vi "Read current data.vi"(8 "error in":errorcluster) -> (0 "error out":errorcluster, 1 "timestamp":timestamp, 2 "Data Array":T1[](array[typedef]), 3 "Variable Descriptions":T2[](array[typedef]))   [LabVIEW 2017, in "DTACQ - Network Enabled Device Driver.lvlib"]
uses:
  DTACQ - Network Enabled Device Driver.lvlib
  Network Shared Variables/Typedefs/Shared Variable Properties--Cluster.ctl
  Network Shared Variables/Typedefs/X and Y Variant Arrays--Cluster.ctl
  Network Shared Variables/Shared Variables Library.lvlib
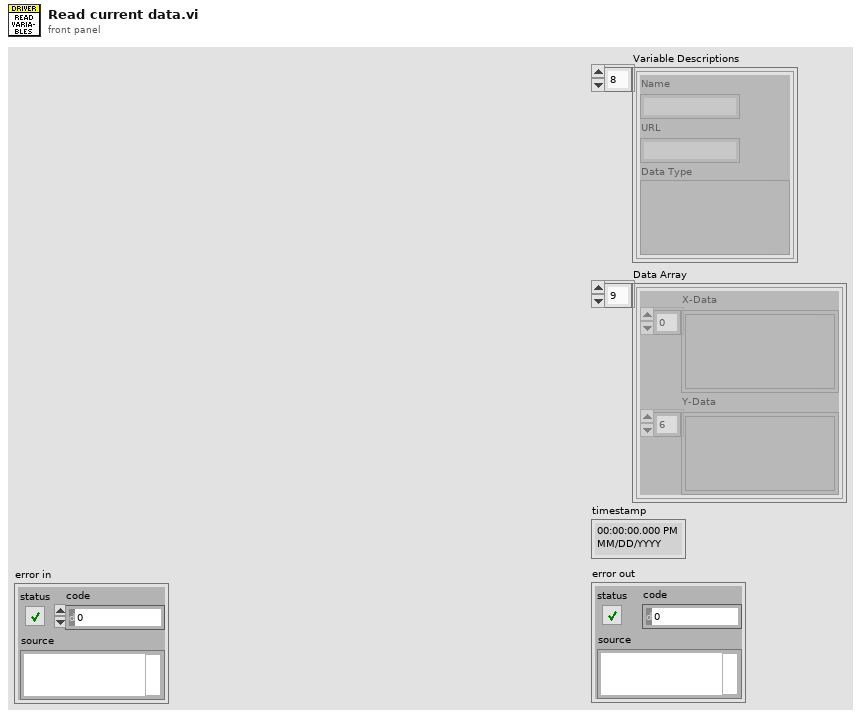
[diagram p1: front panel]
types:
  T1 = typedef "Shared Variables Library.lvlib/X and Y Variant Arrays--Cluster.ctl" = cluster{"X-Data":variant[], "Y-Data":variant[]}
  T2 = typedef "Shared Variables Library.lvlib/Shared Variable Properties--Cluster.ctl" = cluster{"Name":string, "URL":string, "Data Type":variant}
  T3 = cluster{"Read Access":enum8{"Allowed", "Required", "None"}, "Write Access":enum8{"Allowed", "Required", "None"}}
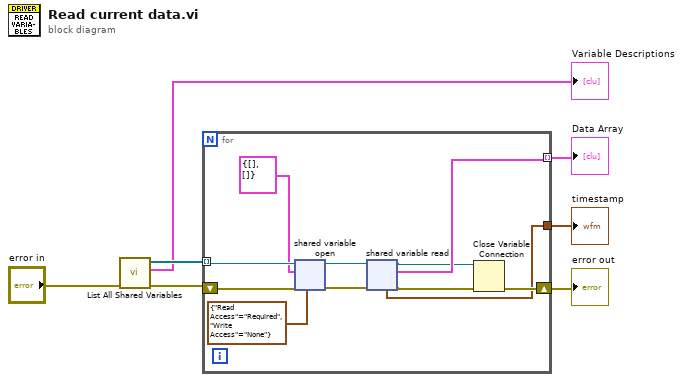
[diagram p0: block diagram]
diagram:
  n1 = call "List All Shared Variables.vi"("error in"="error in") -> ("error out"=w3:errorcluster, "Variable Descriptions"=→"Variable Descriptions":T2[], "Variable References"=w7:refnum<k21>[])  [unwired: 8 in]
  n2 = for {
    tunnel: w7 -> [w18] mode=indexing
    shift-right: [w15] -> w6
    shift-left: w3 -> [w16]
    tunnel: [w12] -> w4 mode=indexing
    tunnel: [w8] -> w1
    n3 = shared-variable-open(w18, w16, T1 {"X-Data"=[], "Y-Data"=[]} ("Data Cluster"), T3 {"Read Access"=enum."Required", "Write Access"=enum."None"} ("access")) -> (w13:refnum<k21>, w14:errorcluster)
    n4 = shared-variable-read(w13, w14) -> (w10:refnum<k21>, w11:errorcluster, w12:T1, w8:timestamp)
    n5 = Close Variable Connection(8:w11, 11:w10) -> (0:w15:errorcluster)
  }
  "error out" <- w6
  "Data Array" <- w4
  "timestamp" <- w1
